vi "Array Teil gesamt.vi"(8 "Spalten":i32, 9 "Zeilen":i32=1, 10 "Key":string, 11 "Data":string[][](array[string])) -> (2 "Data Part (Ausgang)":string[][](array[string]), 3 "Teil Array (Ausgang)":string[][](array[string]))   [LabVIEW 2020, in "Linearisierung v2.lvlib"]
uses:
  Linearisierung v2.lvlib
  SpanEinstellungen/SpanEinstellungen.lvlib
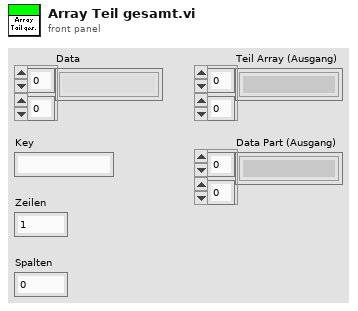
[diagram p1: front panel]
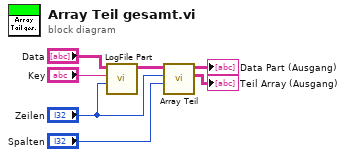
[diagram p0: block diagram]
diagram:
  n1 = call "LogFile Part.vi"("Länge"="Zeilen", "Key"="Key", "Data"="Data") -> ("Part Array"=w7:string[][])  [unwired: 8 in]
  n2 = call "Array Teil.vi"("Spalten"="Spalten", "Zeilen"="Zeilen", "Array (Eingang)"=w7) -> ("Teil Array (Ausgang)"=→"Teil Array (Ausgang)":string[][], "Array (Ausgang)"=→"Data Part (Ausgang)":string[][])  [unwired: 7 in]
